vi "Err_SizeCheck.vi"(2 "data 2":u8[](array[numeric]), 3 "data":u8[](array[numeric])) -> ()   [LabVIEW 2024]
doc: "This VI checks to see if two images are the same size or not. If the images are not the same size, it throws an error message to the user."
uses:
  <userlib>/ImageProcessing/CameraGlobals.vi
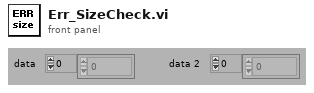
[diagram p1: front panel]
types:
  T1 = typedef "QT_Ref.ctl" = refnum<k1>
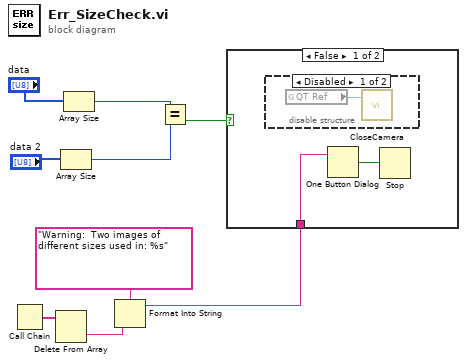
[diagram p0: block diagram]
diagram:
  n1 = Call Chain() -> (call chain=w8:string[])
  n2 = Delete From Array(array=w8) -> (deleted portion=w7:string)  [unwired: 2 in, 1 out]
  n3 = Array Size(array="data 2") -> (size(s)=w2:i32)
  n4 = Array Size(array="data") -> (size(s)=w3:i32)
  n5 = Format Into String(format string="Warning:  Two images of different sizes used in: %s" ("message"), w7) -> (resulting string=w6:string)  [unwired: 2 in, 1 out]
  n6 = Equal?(x=w3, y=w2) -> (x = y?=w1:bool)
  n7 = case shown="False" w1 {
    tunnel: w6 -> [w11 _]
    frame False {
      n8 = disable-structure shown="Disabled" {
        frame Disabled {
          n9 = global read "CameraGlobals.vi" "QT Ref"() -> (w12:T1)
          n10 = call <userlib>:"CloseCamera.vi"("QT Ref In"=w12) -> ()  [unwired: 2 in, 1 out]
        }
        frame Enabled {
        }
      }
      n11 = One Button Dialog(message=w11) -> (true=w10:bool)  [unwired: 1 out]
      n12 = Stop(stop? (T)=w10) -> ()
    }
    frame True {
    }
  }
